vi "BaseProvider_GetDesignPatternMethods.vi"(1 "DesignPattern":T1[](array[typedef]), 2 "ClassTemplateName":string, 3 "ConnectorPaneSettings":string, 5 "error in":errorcluster) -> (15 "NormalMethods":T3[](array[typedef]), 19 "error out":errorcluster)   [LabVIEW 2016]
uses:
  <resource>/Framework/Providers/Open_GDS/ClassProviders/Provider_LvNativeClass/ClassWriterNative_class/MethodInfo.ctl
  <resource>/Framework/Providers/Open_GDS/ClassProviders/Provider_LvNativeClass/ClassWriterNative_class/MethodType.ctl
  <resource>/Framework/Providers/Open_GDS/ClassProviders/Common/LvClass_class/GDSLvClass_PlugIn.ctl
  <resource>/Framework/Providers/Open_GDS/ClassProviders/Common/LvClass_class/GDSLvClass_PlugInTypes.ctl
  <vilib>/Utility/config.llb/Read Key (String).vi
  <vilib>/Utility/config.llb/NI_LVConfig.lvlib
  <resource>/Framework/Providers/Open_GDS/ClassProviders/Provider_LvNativeClass/ClassWriterNative_class/ClassWriterNative.lvclass
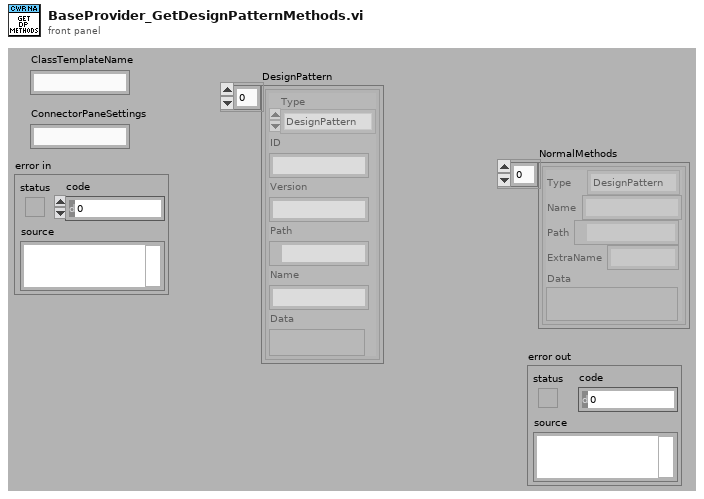
[diagram p1: front panel]
types:
  T1 = typedef "GDSLvClass_PlugIn.ctl" = cluster{"Type":T2, "ID":string, "Version":string, "Path":path, "Name":string, "Data":variant}
  T2 = typedef "GDSLvClass_PlugInTypes.ctl" = enum16{"DesignPattern", "MethodTypes"}
  T3 = typedef "ClassWriterNative.lvclass/MethodInfo.ctl" = cluster{"Type":T4, "Name":string, "Path":path, "ExtraName":string, "Data":variant}
  T4 = typedef "ClassWriterNative.lvclass/MethodType.ctl" = enum16{"Normal", "MethodPlugIn", "DesignPattern", "AF-Method"}
  T5 = typedef "NI_LVConfig.lvlib/Config Data RefNum.ctl" = refnum<k1>
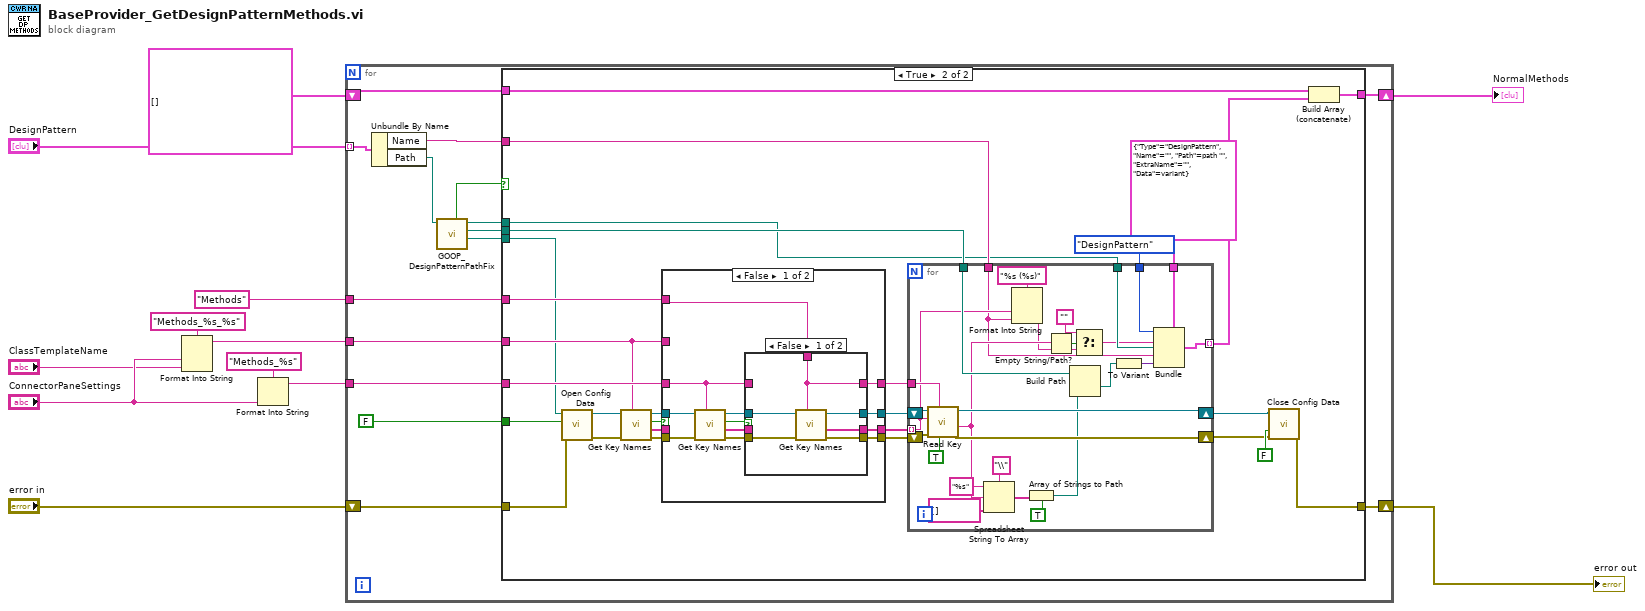
[diagram p0: block diagram]
diagram:
  n1 = Format Into String(format string="Methods_%s_%s" ("section"), "ConnectorPaneSettings", "ClassTemplateName") -> (resulting string=w2:string)  [unwired: 2 in, 1 out]
  n2 = Format Into String(format string="Methods_%s" ("section"), "ConnectorPaneSettings") -> (resulting string=w6:string)  [unwired: 2 in, 1 out]
  n3 = for {
    shift-right: [w17] -> w11
    shift-left: "error in" -> [w27]
    tunnel: "DesignPattern" -> [w25] mode=indexing
    shift-right: [w23] -> w8
    shift-left: T3[] [] ("NormalMethods") -> [w24]
    tunnel: w6 -> [w20]
    tunnel: w2 -> [w18]
    tunnel: "Methods" ("section") -> [w19]
    n4 = Unbundle By Name(w25) -> ("Name"=w22:string, "Path"=w15:path)
    n5 = call <resource>:"GOOP_DesignPatternPathFix.vi"("ViPathIn"=w15) -> ("Ini-File"=w16:path, "Folder"=w21:path, "ViPathOut"=w14:path, "Found"=w13:bool)  [unwired: 6 in, 1 out]
    n6 = case shown="True" w13 {
      tunnel: w27 -> [w29 w57]
      tunnel: FALSE ("create file if necessary? (T)") -> [_ w55]
      tunnel: w24 -> [w28 w49]
      tunnel: [w28 w47] -> w23
      tunnel: w22 -> [_ w44]
      tunnel: w21 -> [_ w43]
      tunnel: w20 -> [_ w41]
      tunnel: w19 -> [_ w34]
      tunnel: w18 -> [_ w33]
      tunnel: [w29 w32] -> w17
      tunnel: w16 -> [_ w31]
      tunnel: w14 -> [_ w30]
      frame False {
      }
      frame True {
        n7 = call <vilib>:"Open Config Data.vi"("error in (no error)"=w57, "create file if necessary (T)"=w55, "configuration file path"=w31) -> ("error out"=w40:errorcluster, "refnum"=w39:T5)  [unwired: 6 in, 1 out]
        n8 = call <vilib>:"Get Key Names.vi"("section"=w33, "error in (no error)"=w40, "refnum"=w39) -> ("error out"=w38:errorcluster, "key names"=w35:string[], "section exists?"=w36:bool, "refnum out"=w37:T5)  [unwired: 5 in]
        n9 = case shown="False" w36 {
          tunnel: [w69 w83] -> w54
          tunnel: [w68 w82] -> w53
          tunnel: [w67 w81] -> w52
          tunnel: [w62 w80] -> w42
          tunnel: w41 -> [w61 _]
          tunnel: w38 -> [w60 w81]
          tunnel: w37 -> [w59 w82]
          tunnel: w35 -> [_ w83]
          tunnel: w34 -> [w58 _]
          tunnel: w33 -> [_ w80]
          frame False {
            n10 = call <vilib>:"Get Key Names.vi"("section"=w61, "error in (no error)"=w60, "refnum"=w59) -> ("error out"=w64:errorcluster, "key names"=w63:string[], "section exists?"=w65:bool, "refnum out"=w66:T5)  [unwired: 5 in]
            n11 = case shown="False" w65 {
              tunnel: [w75 w79] -> w69
              tunnel: [w74 w78] -> w68
              tunnel: [w73 w77] -> w67
              tunnel: w66 -> [w72 w78]
              tunnel: w64 -> [w71 w77]
              tunnel: w63 -> [_ w79]
              tunnel: [w70 w76] -> w62
              tunnel: w61 -> [_ w76]
              tunnel: w58 -> [w70 _]
              frame False {
                n12 = call <vilib>:"Get Key Names.vi"("section"=w70, "error in (no error)"=w71, "refnum"=w72) -> ("error out"=w73:errorcluster, "key names"=w75:string[], "refnum out"=w74:T5)  [unwired: 5 in, 1 out]
              }
              frame True {
              }
            }
          }
          frame True {
          }
        }
        n13 = for {
          shift-right: [w103] -> w50
          shift-left: w52 -> [w109]
          shift-right: [w104] -> w51
          shift-left: w53 -> [w110]
          tunnel: w42 -> [w108]
          tunnel: w54 -> [w87] mode=indexing
          tunnel: [w99] -> w48 mode=indexing
          tunnel: w43 -> [w105]
          tunnel: T3 {"Type"=enum."DesignPattern", "Name"="", "Path"=path "", "ExtraName"="", "Data"=variant} ("Cluster") -> [w102]
          tunnel: MethodType."DesignPattern" ("Type") -> [w101]
          tunnel: w30 -> [w100]
          tunnel: w44 -> [w86]
          n14 = call-poly <vilib>:"Read Key.vi"("read raw string? (F)"=TRUE, "section"=w108, "error in (no error)"=w109, "key"=w87, "refnum"=w110) -> ("error out"=w103:errorcluster, "value"=w90:string, "refnum out"=w104:T5)  [unwired: 3 in, 1 out]
          n15 = Spreadsheet String To Array(delimiter (Tab)="\\", format string="%s", spreadsheet string=w90, array type (2D Dbl)=string[] []) -> (array=w91:string[])
          n16 = Format Into String(format string="%s (%s)", w87, w86) -> (resulting string=w84:string)  [unwired: 2 in, 1 out]
          n17 = Array of Strings to Path(0:w91, 1:TRUE ("relative")) -> (2:w89:path)
          n18 = Empty String/Path?(string/path=w90) -> (empty?=w107:bool)
          n19 = Build Path(base path=w105, name or relative path=w89) -> (appended path=w98:path)
          n20 = Select(t="", s=w107, f=w84) -> (s? t:f=w97:string)
          n21 = To Variant(anything=w98) -> (Variant=w88:variant)
          n22 = Bundle(cluster=w102, "Type"=w101, "Name"=w97, "Path"=w100, "ExtraName"=w86, "Data"=w88) -> (w99:T3)
        }
        n23 = call <vilib>:"Close Config Data.vi"("error in (no error)"=w50, "write file if changed (T)"=FALSE ("create file if necessary? (T)"), "refnum"=w51) -> ("error out"=w32:errorcluster)  [unwired: 7 in, 1 out]
        n24 = Build Array (concatenate)(w49, w48) -> (w47:T3[])
      }
    }
  }
  "NormalMethods" <- w8
  "error out" <- w11
